vi "BUtton - DIR Trans.vi"(0 "Direction":T1(ring)) -> (1 "Front":bool, 2 "Left":bool, 3 "Right":bool, 4 "Back":bool)   [LabVIEW 2015]
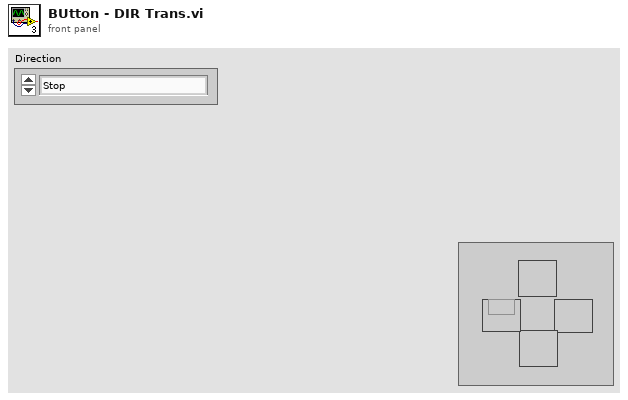
[diagram p1: front panel]
types:
  T1 = enum16{"Stop", "Front", "FR", "Right", "BR", "Back", "BL", "Left", "FL"}
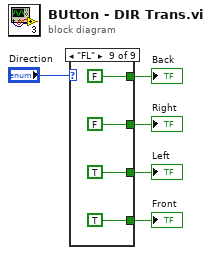
[diagram p0: block diagram]
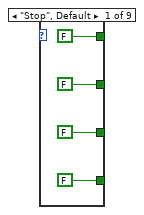
[diagram p2: hidden frame]
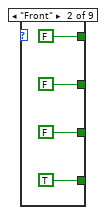
[diagram p3: hidden frame]
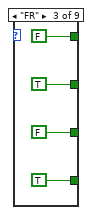
[diagram p4: hidden frame]
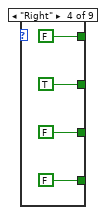
[diagram p5: hidden frame]
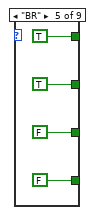
[diagram p6: hidden frame]
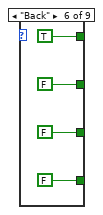
[diagram p7: hidden frame]
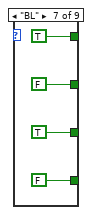
[diagram p8: hidden frame]
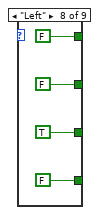
[diagram p9: hidden frame]
diagram:
  n1 = case shown="\"FL\"" "Direction" {
    tunnel: [FALSE TRUE TRUE FALSE FALSE FALSE FALSE FALSE TRUE] -> w5
    tunnel: [FALSE FALSE TRUE TRUE TRUE FALSE FALSE FALSE FALSE] -> w4
    tunnel: [FALSE FALSE FALSE FALSE TRUE TRUE TRUE FALSE FALSE] -> w3
    tunnel: [FALSE FALSE FALSE FALSE FALSE FALSE TRUE TRUE TRUE] -> w2
    frame "Stop", Default {
    }
    frame "Front" {
    }
    frame "FR" {
    }
    frame "Right" {
    }
    frame "BR" {
    }
    frame "Back" {
    }
    frame "BL" {
    }
    frame "Left" {
    }
    frame "FL" {
    }
  }
  "Left" <- w2
  "Back" <- w3
  "Right" <- w4
  "Front" <- w5
